vi "8.4-Test of Lead Controller.vi"() -> ()   [LabVIEW 2010]
panel:
  in  "Input K s14fxp-6":fxp<+/-,14,-6> format="%.19e"
  in  "Input C u8fxp-2":fxp<+,8,-2> format="%b"
  out "Waveform Graph":dbl[](graph)
  out "Array 2":dbl[][](array[numeric])
  in  "Error Array":i32[](array[numeric])
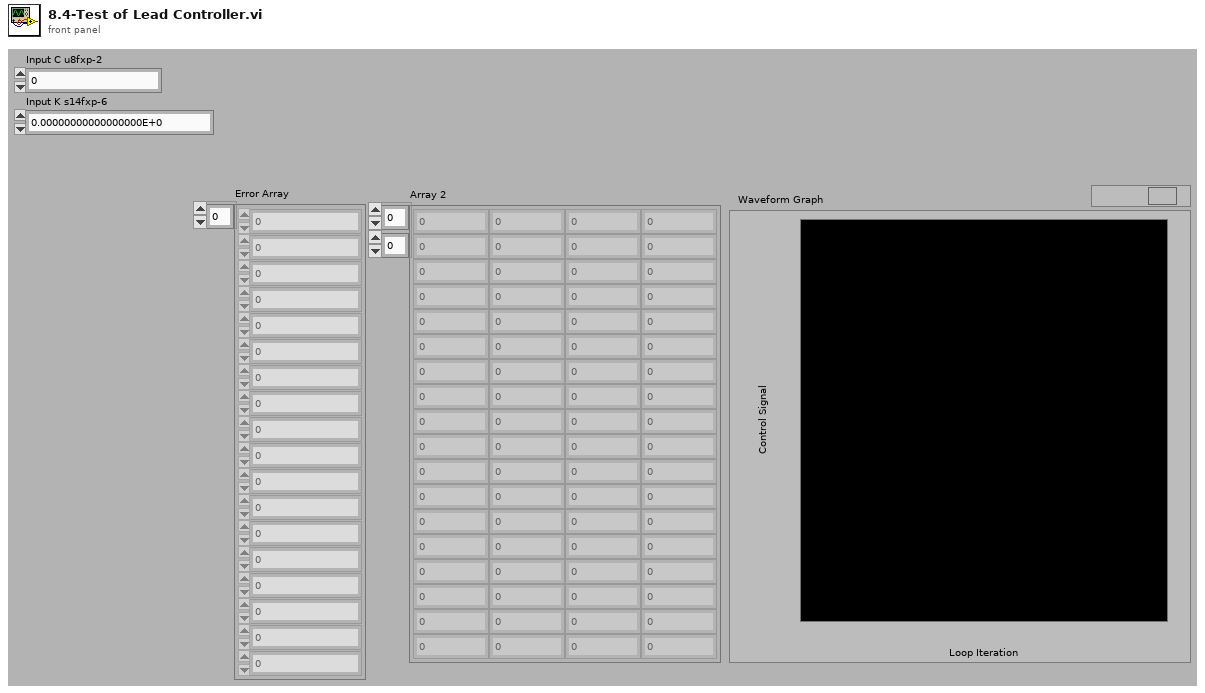
[diagram p1: front panel]
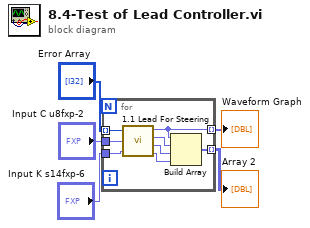
[diagram p0: block diagram]
diagram:
  n1 = for {
    tunnel: "Error Array" -> [w13] mode=indexing
    tunnel: "Input C u8fxp-2" -> [w12]
    tunnel: "Input K s14fxp-6" -> [w11]
    tunnel: [w10] -> w1 mode=indexing
    tunnel: [w6] -> w2 mode=indexing
    n2 = call "1.1 Lead For Steering.vi"("Input K s14fxp-6"=w11, "Input C u8fxp-2"=w12, "Error Input"=w13) -> ("s(sqrt(10)s+bdt)/(s/sqrt(10)+bdt)"=w7:fxp<+/-,20,22>, "(sqrt(10)s+bdt)/(s/sqrt(10)+bdt)"=w8:fxp<+/-,20,22>, "sqrt(10)s+bdt"=w9:fxp<+/-,18,20>, "Controls Output"=w10:fxp<+/-,20,5>)
    n3 = Build Array(w10, w9, w8, w7) -> (w6:fxp<+/-,37,22>[])
  }
  "Array 2" <- w2
  "Waveform Graph" <- w1
